vi "Msg.vi"(7 "Queue Actor in":refnum<class "Queue Actor.lvclass">, 11 "Pop Up Msg in":refnum<class "Pop Up Msg.lvclass">) -> (5 "Queue Actor out":refnum<class "Queue Actor.lvclass">)   [LabVIEW 2021, in "Pop Up.lvlib" / "Pop Up Msg.lvclass"]
uses:
  Pop Up Msg.lvclass
  Actor/Queue Actor/Queue Actor.lvclass
  Pop Up/Pop Up.lvclass
  c6b198b1-1ebb-4276-964f-c3ad762143cc.vi
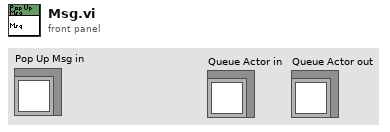
[diagram p1: front panel]
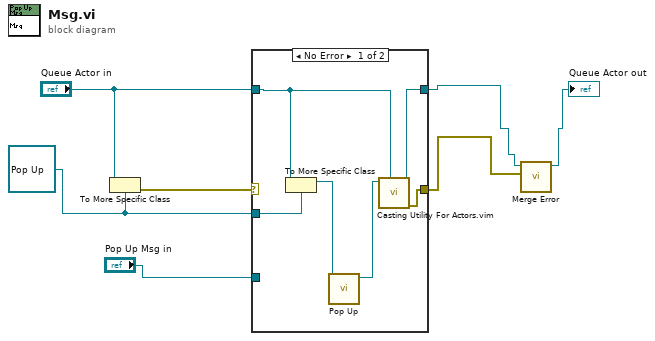
[diagram p0: block diagram]
diagram:
  w5 = refnum<class "Pop Up.lvclass"> refnum ("Pop Up.lvlib:Pop Up.lvclass")
  n1 = To More Specific Class(target class=w5, reference="Queue Actor in") -> (error out=w7:errorcluster)  [unwired: 1 in, 1 out]
  n2 = case shown="No Error" w7 {
    selector: w7 -> [_ w14]
    tunnel: [w12 w15] -> w3
    tunnel: "Queue Actor in" -> [w8 w15]
    tunnel: w5 -> [w13 _]
    tunnel: "Pop Up Msg in" -> [_ _]
    tunnel: [w11 w14] -> w1
    frame No Error {
      n3 = To More Specific Class(target class=w13, reference=w8) -> (specific class reference=w10:refnum<class "Pop Up.lvclass">)  [unwired: 1 in, 1 out]
      n4 = call-dynamic "Pop Up.vi"("Pop Up in"=w10) -> ("Pop Up out"=w9:refnum<class "Pop Up.lvclass">)  [unwired: 10 in]
      n5 = call "Casting Utility For Actors.vim"("type"=w8, "Actor in"=w9) -> ("error out"=w11:errorcluster, "Actor out"=w12:refnum<class "Queue Actor.lvclass">)  [unwired: 8 in]
    }
    frame Error {
    }
  }
  n6 = call-dynamic "Merge Error.vi"("Error"=w1, "Set Error in"=w3) -> ("Set Error out"=→"Queue Actor out":refnum<class "Queue Actor.lvclass">)  [unwired: 9 in]
